vi "Convert Data Type String to Data Type Code - Single Input.vi"(8 "Error In":errorcluster, 11 "Type":string) -> (0 "Error Out":errorcluster, 2 "Type code":i32, 3 "Type":string)   [LabVIEW 2014]
doc: "<B>Copyright</B>: (c) MHWirth 2015.\n\nThis VI converts the array of data types (string) to array of data type codes (int32). \n\n<B>Defined Type Code</B>:\nUnknown/Undefined type returns -1. \nCode 1. Boolean\nCode 2 to 5. Int8/16/32/64\nCode 6 to 9. UInt8/16/32/64\nCode 10. Double\nCode 11. Single-precision\nCode 12. String\nCode 13 to 24. 1D array of xxx\nCode 25 to 36. 2D array of xxx"
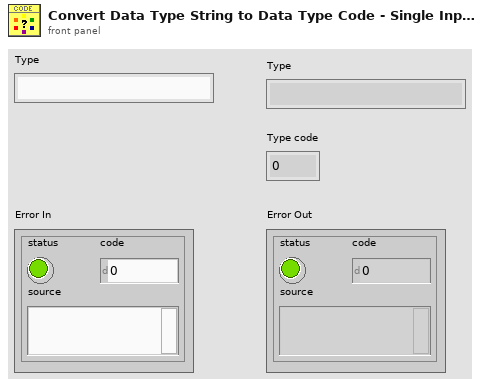
[diagram p1: front panel]
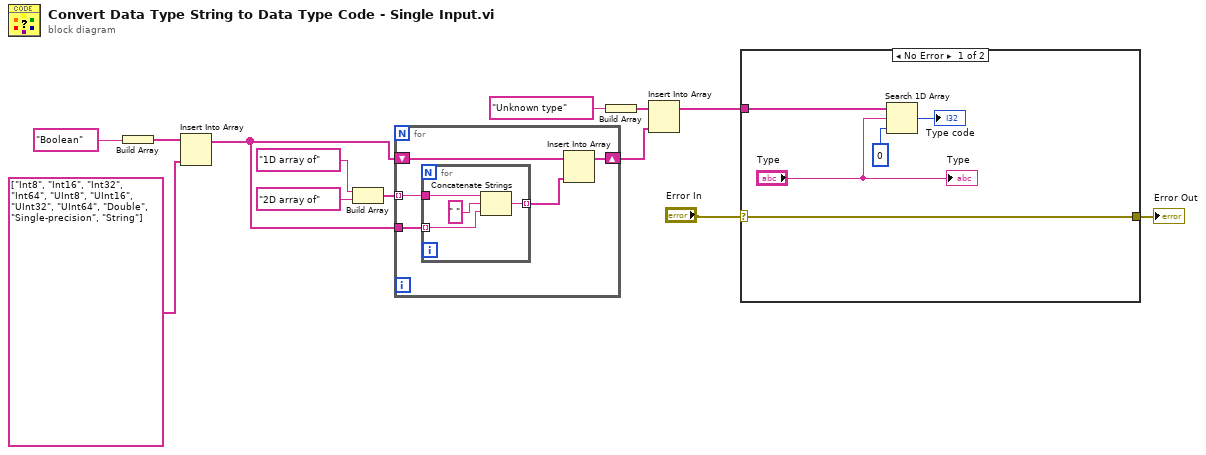
[diagram p0: block diagram]
diagram:
  n1 = Build Array("Boolean") -> (w3:string[])
  n2 = Insert Into Array(array=w3, new element=string[] ["Int8", "Int16", "Int32", "Int64", "UInt8", "UInt16", "UInt32", "UInt64", "Double", "Single-precision", "String"]) -> (w1:string[])  [unwired: 1 in]
  n3 = Build Array("1D array of", "2D array of") -> (w9:string[])
  n4 = for {
    tunnel: w9 -> [w18] mode=indexing
    shift-right: [w15] -> w8
    shift-left: w1 -> [w17]
    tunnel: w1 -> [w14]
    n5 = for {
      tunnel: w18 -> [w22]
      tunnel: w14 -> [w20] mode=indexing
      tunnel: [w19] -> w16 mode=indexing
      n6 = Concatenate Strings(w22, " ", w20) -> (w19:string)
    }
    n7 = Insert Into Array(array=w17, new element=w16) -> (w15:string[])  [unwired: 1 in]
  }
  n8 = Build Array("Unknown type") -> (w6:string[])
  n9 = Insert Into Array(array=w6, new element=w8) -> (w5:string[])  [unwired: 1 in]
  n10 = case shown="No Error" "Error In" {
    selector: "Error In" -> [w27 w28]
    tunnel: [w27 w28] -> w12
    tunnel: w5 -> [w26 _]
    frame No Error {
      n11 = Search 1D Array(1D array=w26, element="Type", start index (0)=0) -> (index of element=→"Type code":i32)
      "Type" <- "Type"
    }
    frame Error {
    }
  }
  "Error Out" <- w12
